vi "SV Buffer Waveform (No State) (DBL).vi"(7 "clear buffer (False)":bool, 8 "error in (no error)":errorcluster, 9 "buffer length [s] (-1 = unlimited)":dbl=-1.0, 10 "waveform":waveform(dbl), 11 "buffer in":waveform(dbl)) -> (0 "error out":errorcluster, 3 "buffer out":waveform(dbl))   [LabVIEW 2017]
uses:
  <vilib>/addons/_NISVFA/_Shared subVIs/Controls/svc_Waveform Parameters.ctl
  <vilib>/addons/_NISVFA/_Shared subVIs/Common/svc_Get Array Subset (Index).vi
  <vilib>/addons/_NISVFA/_Shared subVIs/Common/svc_Get SV Channel Info.vi
  <vilib>/addons/_NISVFA/_Shared subVIs/Common/svc_Coerce Index and Length.vi
  <vilib>/addons/_NISVFA/_Shared subVIs/Common/svc_Conditional Merge Error.vi
  <vilib>/addons/_NISVFA/_Shared subVIs/Common/svc_Engineering Units to Unit Label.vi
  <vilib>/addons/_NISVFA/_Shared subVIs/Common/svc_Unit Label to Engineering Units.vi
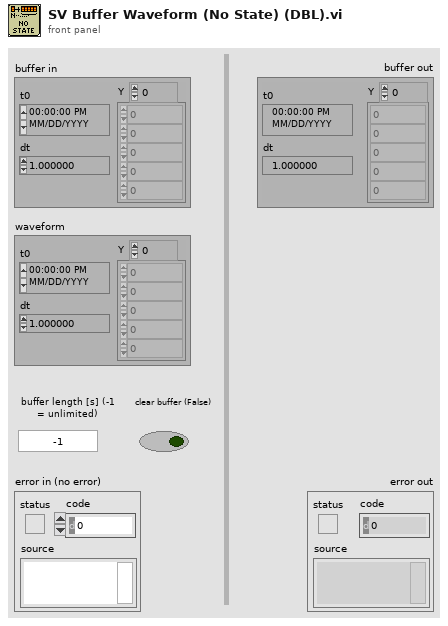
[diagram p1: front panel]
types:
  T1 = typedef "svc_Waveform Parameters.ctl" = cluster{"channel name":string, "t0":timestamp, "dt":dbl, "array length":i32}
  T2 = cluster{"dt":bool, "t0 continuity":bool, "array length":bool, "channel info":bool, "name":bool}
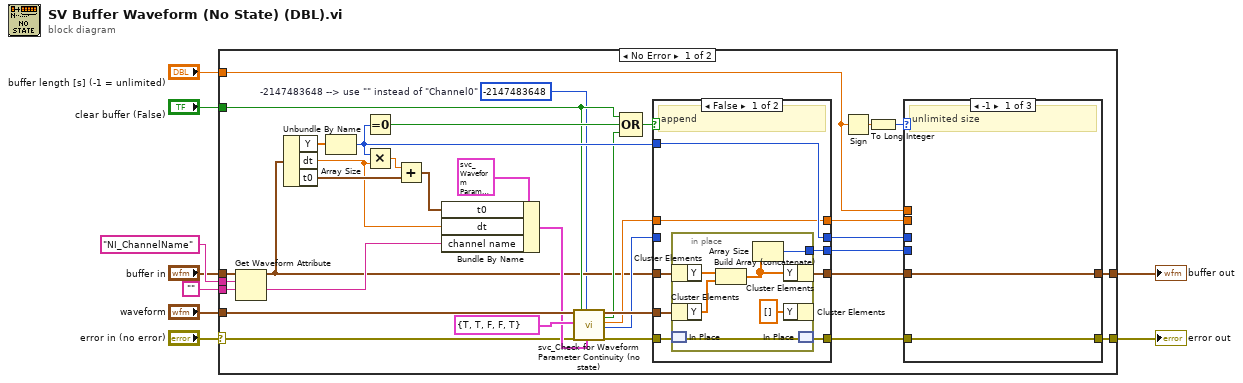
[diagram p0: block diagram]
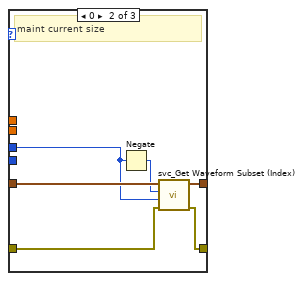
[diagram p2: hidden frame]
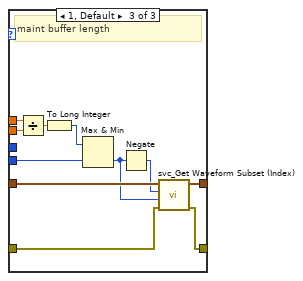
[diagram p3: hidden frame]
diagram:
  n1 = case shown="No Error" "error in (no error)" {
    selector: "error in (no error)" -> [w16 w82]
    tunnel: [w42 w83] -> w9
    tunnel: "buffer length [s] (-1 = unlimited)" -> [w12 _]
    tunnel: "clear buffer (False)" -> [w35 _]
    tunnel: "waveform" -> [w33 _]
    tunnel: "NI_ChannelName" ("name") -> [w24 _]
    tunnel: "buffer in" -> [w23 w83]
    tunnel: "" -> [w22 _]
    tunnel: [w17 w82] -> w2
    frame No Error {
      w15 = -2147483648  # -2147483648 --> use "" instead of "Channel0"
      n2 = Get Waveform Attribute(5:w22, 6:w24, 7:w23) -> (1:w21:string, 3:w20:waveform(dbl))  [unwired: 1 in, 2 out]
      n3 = Unbundle By Name(w20) -> ("Y"=w41:dbl[], "dt"=w25:dbl, "t0"=w37:timestamp)
      n4 = Array Size(array=w41) -> (size(s)=w38:i32)
      n5 = Equal To 0?(x=w38) -> (x = 0?=w40:bool)
      n6 = Multiply(x=w38, y=w25) -> (x*y=w36:dbl)
      n7 = Add(x=w36, y=w37) -> (x+y=w26:timestamp)
      n8 = Bundle By Name(cluster=T1 {"channel name"="", "t0"=timestamp(0 s since 1904-01-01), "dt"=0.0, "array length"=0} ("expected waveform parameters"), "t0"=w26, "dt"=w25, "channel name"=w21) -> (w27:T1)
      n9 = call <vilib>:"svc_Check for Waveform Parameter Continuity (no state).vi"("scaled signal [EU]"=w33, "checks for channel parameter change"=T2 {"dt"=TRUE, "t0 continuity"=TRUE, "array length"=FALSE, "channel info"=FALSE, "name"=TRUE}, "error in (no error)"=w16, "reset"=w35, "channel index"=w15, "expected waveform parameters"=w27) -> ("dup scaled signal [EU]"=w32:waveform(dbl), "waveform parameter changed"=w29:bool, "dt"=w30:dbl, "array length"=w31:i32, "error out"=w19:errorcluster)  [unwired: 7 in, 2 out]
      n10 = Compound Arithmetic op=OR(w35, w40, w29) -> (w39:bool)
      n11 = case shown="False" w39 {
        tunnel: w20 -> [w69 _]
        tunnel: w32 -> [w66 w81]
        tunnel: [w70 w80] -> w11
        tunnel: [w71 w78] -> w43
        tunnel: [w65 w81] -> w44
        tunnel: w31 -> [_ w78]
        tunnel: w38 -> [w71 _]
        tunnel: w30 -> [w70 w80]
        tunnel: w19 -> [w68 w79]
        tunnel: [w67 w79] -> w18
        tunnel: [w64 w78] -> w10
        frame False {
          # "append"
          n12 = in-place {
            in-place-border: [w72] -> w64
            n13 = in-place-cluster #1(w69) -> ("Y"=w76:dbl[])
            n14 = in-place-cluster #2(w66) -> ("Y"=w75:dbl[])
            n15 = in-place-match #3(w68) -> (w77:errorcluster)
            n16 = Build Array (concatenate)(w76, w75) -> (w73:dbl[])
            n17 = Array Size(array=w73) -> (size(s)=w72:i32)
            n18 = in-place-cluster #1("Y"=w73) -> (w65:waveform(dbl))
            n19 = in-place-cluster #2("Y"=dbl[] []) -> ()  [unwired: 1 out]
            n20 = in-place-match #3(w77) -> (w67:errorcluster)
          }
        }
        frame True {
          # "reset"
        }
      }
      n21 = Sign(1:w12) -> (0:w14:dbl)
      n22 = To Long Integer(number=w14) -> (32bit integer=w13:i32)
      n23 = case shown="-1" w13 {
        tunnel: w43 -> [_ w49 _]
        tunnel: [w46 w50 w62] -> w42
        tunnel: w44 -> [w46 w52 w63]
        tunnel: w18 -> [w45 w48 w60]
        tunnel: [w45 w47 w59] -> w17
        tunnel: w12 -> [_ _ w58]
        tunnel: w11 -> [_ _ w57]
        tunnel: w10 -> [_ _ w54]
        frame -1 {
          # "unlimited size"
        }
        frame 0 {
          # "maint current size"
          n24 = Negate(x=w49) -> (-x=w51:i32)
          n25 = call <vilib>:"svc_Get Waveform Subset (Index).vi"("error in (no error)"=w48, "length (-1 = all)"=w49, "start index (0)"=w51, "waveform in"=w52) -> ("error out"=w47:errorcluster, "waveform subset"=w50:waveform(dbl))  [unwired: 2 in, 4 out]
        }
        frame 1, Default {
          # "maint buffer length"
          n26 = Divide(x=w58, y=w57) -> (x/y=w56:dbl)
          n27 = To Long Integer(number=w56) -> (32bit integer=w55:i32)
          n28 = Max & Min(x=w55, y=w54) -> (min(x,y)=w53:i32)  [unwired: 1 out]
          n29 = Negate(x=w53) -> (-x=w61:i32)
          n30 = call <vilib>:"svc_Get Waveform Subset (Index).vi"("error in (no error)"=w60, "length (-1 = all)"=w53, "start index (0)"=w61, "waveform in"=w63) -> ("error out"=w59:errorcluster, "waveform subset"=w62:waveform(dbl))  [unwired: 2 in, 4 out]
        }
      }
    }
    frame Error {
    }
  }
  "buffer out" <- w9
  "error out" <- w2
